vi "support.read_and_free_string_at_address.vi"(6 "string_length":u64, 8 "error in (no error)":errorcluster, 11 "string_ptr":u64) -> (0 "error out":errorcluster, 3 "string":string)   [LabVIEW 2020, in "reqwest.lvlib"]
uses:
  reqwest.lvlib
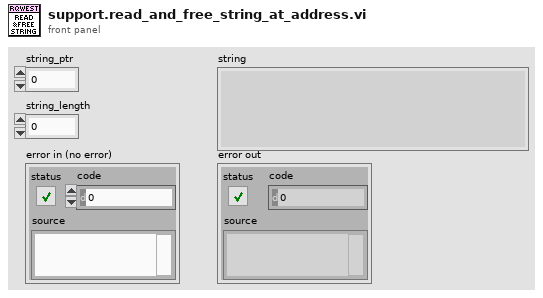
[diagram p1: front panel]
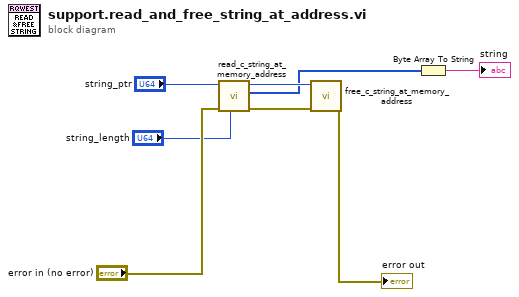
[diagram p0: block diagram]
diagram:
  n1 = call "read_c_string_at_memory_address.vi"("string_length"="string_length", "error in (no error)"="error in (no error)", "memory_address"="string_ptr") -> ("error out"=w7:errorcluster, "data"=w2:u8[], "memory_address out"=w6:u64)  [unwired: 6 in]
  n2 = call "free_c_string_at_memory_address.vi"("error in (no error)"=w7, "memory_address"=w6) -> ("error out"=→"error out":errorcluster)  [unwired: 9 in]
  n3 = Byte Array To String(unsigned byte array=w2) -> (string=→"string":string)
